vi "Generate Two Indices for Local Search.vi"(11 "Schedule in":u16[](array[numeric])) -> (2 "w":i32, 3 "y":i32)   [LabVIEW 2013]
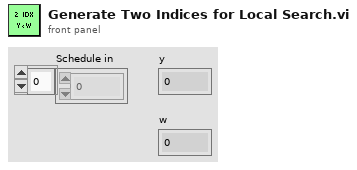
[diagram p1: front panel]
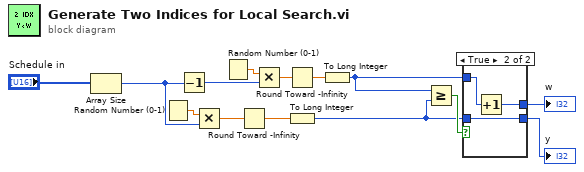
[diagram p0: block diagram]
diagram:
  n1 = Array Size(array="Schedule in") -> (size(s)=w1:i32)
  n2 = Random Number (0-1)() -> (number: 0 to 1=w12:dbl)
  n3 = Decrement(x=w1) -> (x-1=w2:i32)
  n4 = Multiply(x=w12, y=w1) -> (x*y=w11:dbl)
  n5 = Random Number (0-1)() -> (number: 0 to 1=w9:dbl)
  n6 = Round Toward -Infinity(1:w11) -> (0:w10:dbl)
  n7 = Multiply(x=w9, y=w2) -> (x*y=w8:dbl)
  n8 = Round Toward -Infinity(1:w8) -> (0:w7:dbl)
  n9 = To Long Integer(number=w10) -> (32bit integer=w4:i32)
  n10 = To Long Integer(number=w7) -> (32bit integer=w5:i32)
  n11 = Greater Or Equal?(x=w5, y=w4) -> (x >= y?=w6:bool)
  n12 = case shown="True" w6 {
    tunnel: w5 -> [w16 w19]
    tunnel: [w15 w18] -> w3
    tunnel: w4 -> [w15 w17]
    tunnel: [w16 w17] -> w13
    frame False {
    }
    frame True {
      n13 = Increment(x=w19) -> (x+1=w18:i32)
    }
  }
  "y" <- w13
  "w" <- w3
